vi "SoftLimits.vi"(5 "TPR":dbl=162.974662, 7 "Reverse Feedback Sensor":bool, 8 "Sensor position-rev":dbl(knob) scale=0.0..-1024.0, 9 "Offset-rev":dbl(knob) scale=0.0..1024.0, 10 "Rear angle limit":dbl, 11 "Forward angle limit":dbl) -> (1 "Rear limit":dbl, 2 "Forward limit":dbl)   [LabVIEW 2014]
panel:
  in  "Sensor position":dbl(knob)
  in  "Offset":dbl(knob)
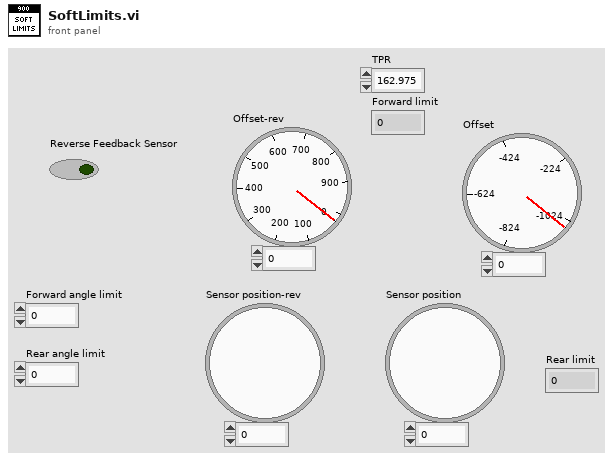
[diagram p1: front panel]
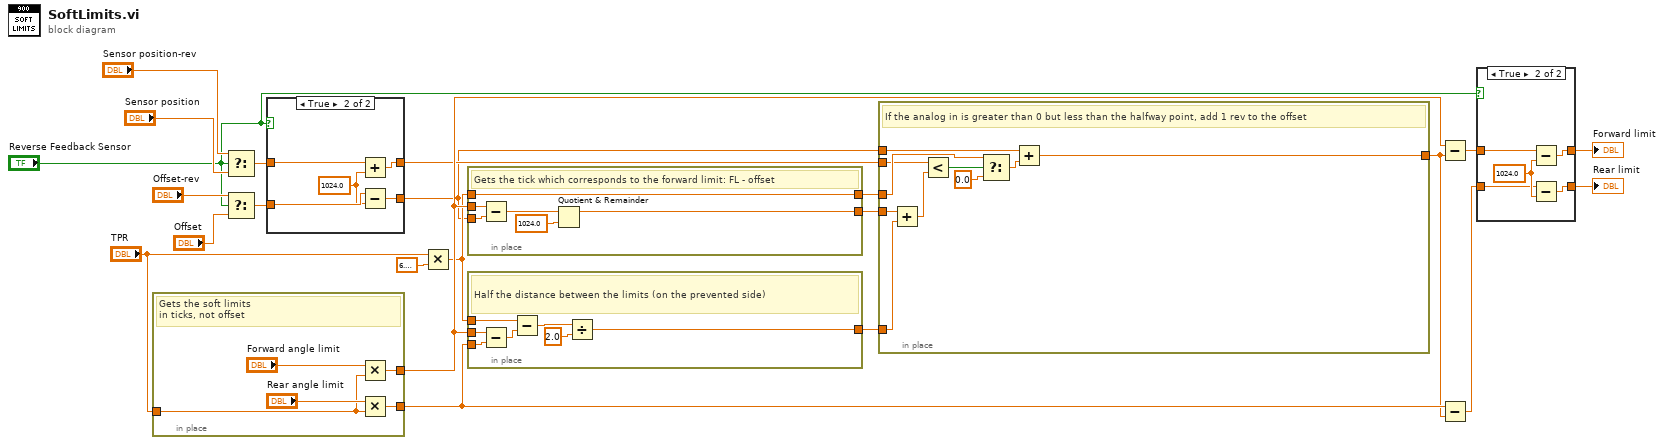
[diagram p0: block diagram]
diagram:
  n1 = in-place {
    in-place-border: "TPR" -> [w25]
    in-place-border: [w24] -> w20
    in-place-border: [w23] -> w19
    # "Gets the soft limits \nin ticks, not offset"
    n2 = Multiply(x="Forward angle limit", y=w25) -> (x*y=w24:dbl)
    n3 = Multiply(x="Rear angle limit", y=w25) -> (x*y=w23:dbl)
  }
  n4 = Select(t="Sensor position-rev", s="Reverse Feedback Sensor", f="Sensor position") -> (s? t:f=w7:dbl)
  n5 = Select(t="Offset-rev", s="Reverse Feedback Sensor", f="Offset") -> (s? t:f=w3:dbl)
  n6 = case shown="True" "Reverse Feedback Sensor" {
    tunnel: [w29 w31] -> w13
    tunnel: w7 -> [w29 w32]
    tunnel: [w28 w33] -> w12
    tunnel: w3 -> [w28 w34]
    frame False {
    }
    frame True {
      w30 = 1024.0 ("y")
      n7 = Add(x=w32, y=w30) -> (x+y=w31:dbl)
      n8 = Subtract(x=w34, y=w30) -> (x-y=w33:dbl)
    }
  }
  n9 = Multiply(x="TPR", y=6.283185307179586) -> (x*y=w14:dbl)
  n10 = in-place {
    in-place-border: [w36] -> w22
    in-place-border: w20 -> [w40]
    in-place-border: w12 -> [w38]
    in-place-border: [w39] -> w17
    in-place-border: w14 -> [w39]
    # "Gets the tick which corresponds to the forward limit: FL - offset"
    n11 = Subtract(x=w40, y=w38) -> (x-y=w37:dbl)
    n12 = Quotient & Remainder(x=w37, y=1024.0) -> (x-y*floor(x/y)=w36:dbl)  [unwired: 1 out]
  }
  n13 = in-place {
    in-place-border: [w45] -> w21
    in-place-border: w20 -> [w44]
    in-place-border: w19 -> [w43]
    in-place-border: w14 -> [w41]
    # "Half the distance between the limits (on the prevented side)"
    n14 = Subtract(x=w44, y=w43) -> (x-y=w47:dbl)
    n15 = Subtract(x=w41, y=w47) -> (x-y=w42:dbl)
    n16 = Divide(x=w42, y=2.0) -> (x/y=w45:dbl)
  }
  n17 = in-place {
    in-place-border: w22 -> [w57]
    in-place-border: w21 -> [w56]
    in-place-border: w12 -> [w54]
    in-place-border: [w52] -> w18
    in-place-border: w17 -> [w51]
    in-place-border: w13 -> [w49]
    # "If the analog in is greater than 0 but less than the halfway point, add 1 rev to the offset"
    n18 = Add(x=w57, y=w56) -> (x+y=w50:dbl)
    n19 = Less?(x=w49, y=w50) -> (x < y?=w48:bool)
    n20 = Select(t=w51, s=w48, f=0.0) -> (s? t:f=w53:dbl)
    n21 = Add(x=w54, y=w53) -> (x+y=w52:dbl)
  }
  n22 = Subtract(x=w20, y=w18) -> (x-y=w10:dbl)
  n23 = Subtract(x=w19, y=w18) -> (x-y=w8:dbl)
  n24 = case shown="True" "Reverse Feedback Sensor" {
    tunnel: [w59 w64] -> w11
    tunnel: w10 -> [w59 w63]
    tunnel: [w58 w61] -> w9
    tunnel: w8 -> [w58 w60]
    frame False {
    }
    frame True {
      w62 = 1024.0 ("x")
      n25 = Subtract(x=w63, y=w62) -> (x-y=w64:dbl)
      n26 = Subtract(x=w60, y=w62) -> (x-y=w61:dbl)
    }
  }
  "Forward limit" <- w11
  "Rear limit" <- w9
